vi "Async Spawn.vi"(4 "Persistent Layers":refnum<class "Actor.lvclass">[](array[class]), 6 "Root":bool, 9 "UID":string, 10 "Unified Actor":refnum<class "Actor.lvclass">, 11 "Core Actor in":refnum<class "Core Actor.lvclass">) -> (0 "Error out":errorcluster, 3 "Core Actor out":refnum<class "Core Actor.lvclass">)   [LabVIEW 2025, in "jettl.lvlib" / "Core Actor.lvlib" / "Core Actor.lvclass"]
uses:
  Core Actor.lvclass
  Actor/Actor.lvclass
  Attributes/Attributes/Attributes.lvclass
  Spawn.ctl
  Async Actor.vi
  Spawn/Spawn/Spawn.lvclass
  Spawn/Spawn.lvlib
  jettl.lvlib
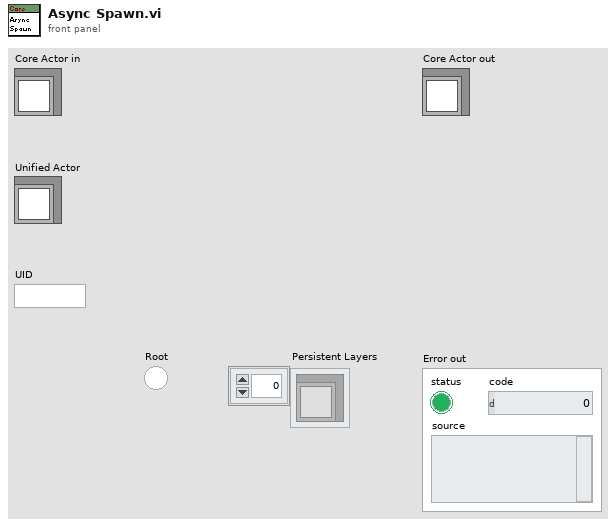
[diagram p1: front panel]
types:
  T1 = typedef "jettl.lvlib/Spawn.ctl" = cluster{"UID":string, "Parent Attributes":refnum<class "Attributes.lvclass">, "Queue of Self Attributes":refnum<queue>, "Queue of Error":refnum<queue>, "Root":bool, "Persistent Layers":refnum<class "Actor.lvclass">[]}
  T2 = typedef "jettl.lvlib/Core Actor.lvlib/Core Actor.lvclass/Child Attributes Map.ctl" = map{string, refnum<class "Attributes.lvclass">}
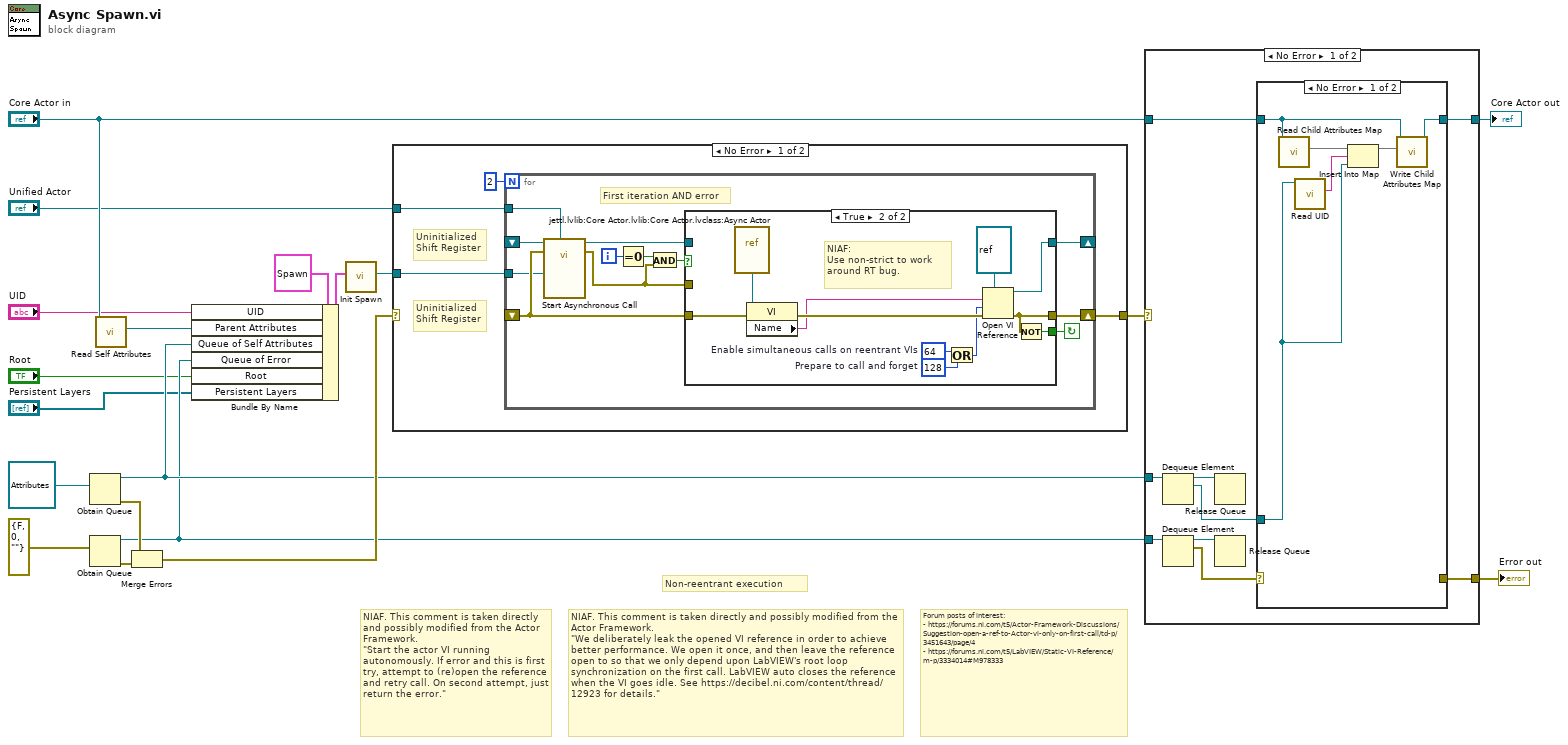
[diagram p0: block diagram]
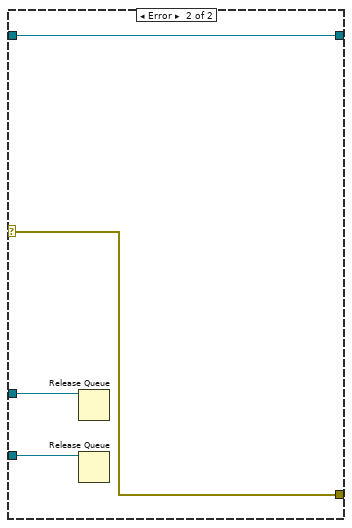
[diagram p3: hidden frame]
diagram:
  # "Forum posts of interest:\n- https://forums.ni.com/t5/Actor-Framework-Discussions/Suggestion-open-a-ref-to-Actor-vi-only-on-first-call/td-p/3451643/page/4\n- https://forums.ni.com/t5/LabVIEW/Static-VI-Reference/m-p/3334014#M978333"
  # "NIAF. This comment is taken directly and possibly modified from the Actor Framework.\n\"We deliberately leak the opened VI reference in order to achieve better performance. We open it once, and then leave the reference open to so that we only depend upon LabVIEW's root loop synchronization on the first call. LabVIEW auto closes the reference when the VI goes idle. See https://decibel.ni.com/content/thread/12923 for details.\""
  # "NIAF. This comment is taken directly and possibly modified from the Actor Framework.\n\"Start the actor VI running autonomously. If error and this is first try, attempt to (re)open the reference and retry call. On second attempt, just return the error.\""
  # "Non-reentrant execution"
  n1 = Obtain Queue(element data type=refnum<class "Attributes.lvclass"> refnum ("jettl.lvlib:Attributes.lvlib:Attributes.lvclass")) -> (queue out=w6:refnum<queue>, error out=w12:errorcluster)  [unwired: 4 in, 1 out]
  n2 = Obtain Queue(element data type=errorcluster {"status"=FALSE, "code"=0, "source"=""} ("Error")) -> (queue out=w5:refnum<queue>, error out=w11:errorcluster)  [unwired: 4 in, 1 out]
  n3 = call-dynamic "Read Self Attributes.vi"("Core Actor in"="Core Actor in") -> ("Self Attributes"=w8:refnum<class "Attributes.lvclass">)  [unwired: 10 in]
  n4 = Merge Errors(w12, w11) -> (w13:errorcluster)
  n5 = Bundle By Name(cluster=T1 {"UID"="", "Parent Attributes"=refnum, "Queue of Self Attributes"=refnum, "Queue of Error"=refnum, "Root"=FALSE, "Persistent Layers"=[]} ("Config Actor"), "UID"="UID", "Parent Attributes"=w8, "Queue of Self Attributes"=w6, "Queue of Error"=w5, "Root"="Root", "Persistent Layers"="Persistent Layers") -> (w4:T1)
  n6 = call "Init Spawn.vi"("Spawn"=w4) -> ("Spawn"=w3:refnum<class "Spawn.lvclass">)  [unwired: 10 in]
  n7 = case shown="No Error" w13 {
    selector: w13 -> [_ w49]
    tunnel: [w20 w49] -> w16
    tunnel: "Unified Actor" -> [w22 _]
    tunnel: w3 -> [w21 _]
    frame No Error {
      # "Uninitialized\nShift Register"
      # "Uninitialized\nShift Register"
      n8 = for {
        N: 2 -> [_]
        shift-right: [w35] -> _
        shift-left: _ -> [w34]
        shift-right: [w32] -> w20
        shift-left: _ -> [w28]
        tunnel: w22 -> [w25]
        tunnel: w21 -> [w24]
        i -> [w30]
        stop <- w29 continue-if-true
        # "First iteration AND error"
        n9 = call-by-ref "Start Asynchronous Call"(reference=w34, error in=w28, "Actor in"=w25, "Spawn"=w24) -> (reference out=w33:refnum<vi>, error out=w26:errorcluster)  [unwired: 8 in, 2 out]
        n10 = Equal To 0?(x=w30) -> (x = 0?=w27:bool)
        n11 = And(x=w27, y=w26) -> (x .and. y?=w31:bool)
        n12 = case shown="True" w31 {
          tunnel: [w37 w46] -> w35
          tunnel: [w36 w44] -> w32
          tunnel: w33 -> [w37 _]
          tunnel: w26 -> [w36 _]
          tunnel: [_ w45] -> w29
          tunnel: w28 -> [_ w43]
          frame False {
          }
          frame True {
            w38 = 64  # Enable simultaneous calls on reentrant VIs
            w40 = 128  # Prepare to call and forget
            # "NIAF:\nUse non-strict to work around RT bug."
            n13 = vi-ref "jettl.lvlib:Core Actor.lvlib:Core Actor.lvclass:Async Actor.vi"() -> (w42:refnum<vi>)
            n14 = property class="VI"(reference=w42, error in=w43) -> (error out=w48:errorcluster, "Name"=w47:string)  [unwired: 1 out]
            n15 = Or(x=w38, y=w40) -> (x .or. y?=w39:i32)
            n16 = Open VI Reference(type specifier VI Refnum (for type only)=refnum<vi> refnum, vi path=w47, options=w39, error in (no error)=w48) -> (vi reference=w46:refnum<vi>, error out=w44:errorcluster)  [unwired: 2 in]
            n17 = Not(x=w44) -> (.not. x?=w45:bool)
          }
        }
      }
    }
    frame Error {
    }
  }
  n18 = case shown="No Error" w16 {
    selector: w16 -> [_ w67]
    tunnel: "Core Actor in" -> [w58 w69]
    tunnel: [w57 w69] -> w19
    tunnel: w6 -> [w56 w70]
    tunnel: w5 -> [w54 w68]
    tunnel: [w50 w67] -> w17
    frame No Error {
      n19 = Dequeue Element(queue=w56) -> (queue out=w55:refnum<queue>, element=w52:refnum<class "Attributes.lvclass">)  [unwired: 2 in, 2 out]
      n20 = Dequeue Element(queue=w54) -> (queue out=w53:refnum<queue>, element=w51:errorcluster)  [unwired: 2 in, 2 out]
      n21 = Release Queue(queue=w55) -> ()  [unwired: 2 in, 3 out]
      n22 = Release Queue(queue=w53) -> ()  [unwired: 2 in, 3 out]
      n23 = case shown="No Error" w51 {
        selector: w51 -> [_ w65]
        tunnel: w58 -> [w63 w66]
        tunnel: [w62 w66] -> w57
        tunnel: w52 -> [w59 _]
        tunnel: [_ w65] -> w50
        frame No Error {
          n24 = call "Read Child Attributes Map.vi"("Core Actor in"=w63) -> ("Child Attributes Map"=w61:T2)  [unwired: 10 in]
          n25 = call-dynamic "Read UID.vi"("Attributes in"=w59) -> ("UID"=w64:string)  [unwired: 10 in]
          n26 = Insert Into Map(map in=w61, key=w64, value=w59) -> (map out=w60:T2)  [unwired: 2 out]
          n27 = call "Write Child Attributes Map.vi"("Child Attributes Map"=w60, "Core Actor in"=w63) -> ("Core Actor out"=w62:refnum<class "Core Actor.lvclass">)  [unwired: 9 in]
        }
        frame Error {
        }
      }
    }
    frame Error {
      n28 = Release Queue(queue=w70) -> ()  [unwired: 2 in, 3 out]
      n29 = Release Queue(queue=w68) -> ()  [unwired: 2 in, 3 out]
    }
  }
  "Core Actor out" <- w19
  "Error out" <- w17
